vi "encoder test box.vi"() -> ()   [LabVIEW 2009]
panel:
  in  "distance in feet":dbl
  in  "stop":bool
  out "error out":errorcluster
  out "Right Encoder Read Dec":u32
  out "Left Encoder Read Dec":u32
  in  "Clear Encoders":bool=TRUE
  in  "MC VISA resource in":refnum<visa-resource-name>="ASRL1::INSTR"
  in  "error in (no error)":errorcluster
  out "MC Init Complete":bool=TRUE
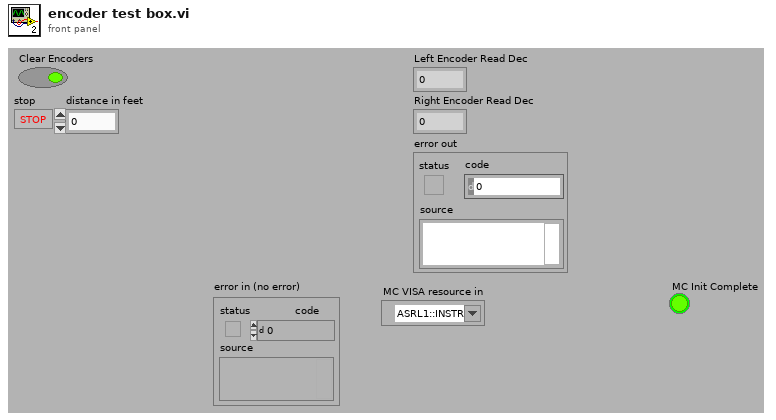
[diagram p1: front panel]
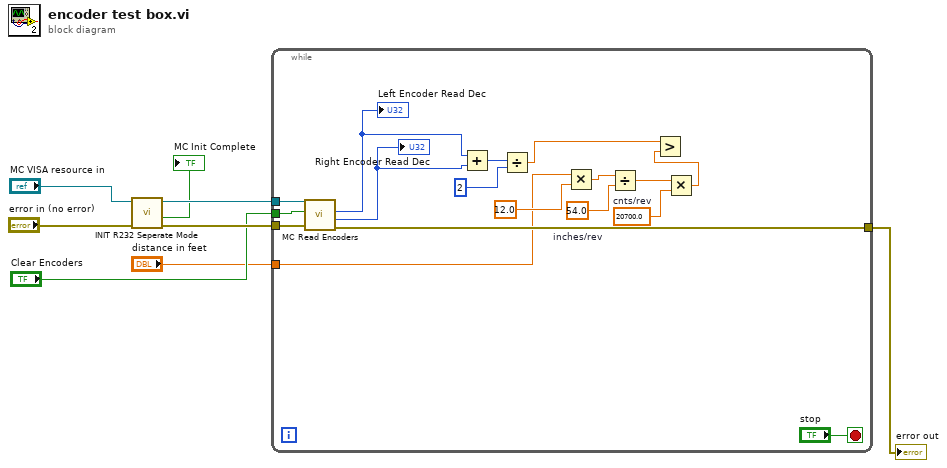
[diagram p0: block diagram]
diagram:
  n1 = call "INIT R232 Seperate Mode.vi"("error in (no error)"="error in (no error)", "MC VISA resource in"="MC VISA resource in") -> ("MC error out"=w6:errorcluster, "MC Init Complete"=→"MC Init Complete":bool, "MC VISA resource  out"=w8:refnum<visa-resource-name>)  [unwired: 7 in]
  n2 = while {
    tunnel: w8 -> [w25]
    tunnel: w6 -> [w24]
    tunnel: "Clear Encoders" -> [w23]
    tunnel: [w22] -> w2
    tunnel: "distance in feet" -> [w10]
    stop <- "stop" stop-if-true
    w11 = 20700.0  # cnts/rev
    w13 = 54.0  # inches/rev
    n3 = call "MC Read Encoders.vi"("error in (no error)"=w24, "Clear Encoders"=w23, "VISA resource name"=w25) -> ("error out"=w22:errorcluster, "Right Encoder Read Dec"=w19:u32, "Left Encoder Read Dec"=w20:u32)  [unwired: 6 in]
    "Left Encoder Read Dec" <- w20
    "Right Encoder Read Dec" <- w19
    n4 = Add(x=w20, y=w19) -> (x+y=w18:u32)
    n5 = Divide(x=w18, y=u32 2) -> (x/y=w16:dbl)
    n6 = Multiply(x=w10, y=12.0) -> (x*y=w14:dbl)
    n7 = Divide(x=w14, y=w13) -> (x/y=w12:dbl)
    n8 = Multiply(x=w12, y=w11) -> (x*y=w9:dbl)
    n9 = Greater?(x=w16, y=w9) -> ()  [unwired: 1 out]
  }
  "error out" <- w2
